vi "Coordinate RND.vi"(8 "error in (no error)":errorcluster, 11 "TSP Class in":refnum<class "TSP Class.lvclass">) -> (0 "error out":errorcluster, 3 "TSP Class out":refnum<class "TSP Class.lvclass">)   [LabVIEW 2015, in "TSP Library.lvlib" / "TSP Class.lvclass"]
uses:
  TSP Class.lvclass
  TSP Class.lvclass/TSP Class.ctl
  TSP Library.lvlib
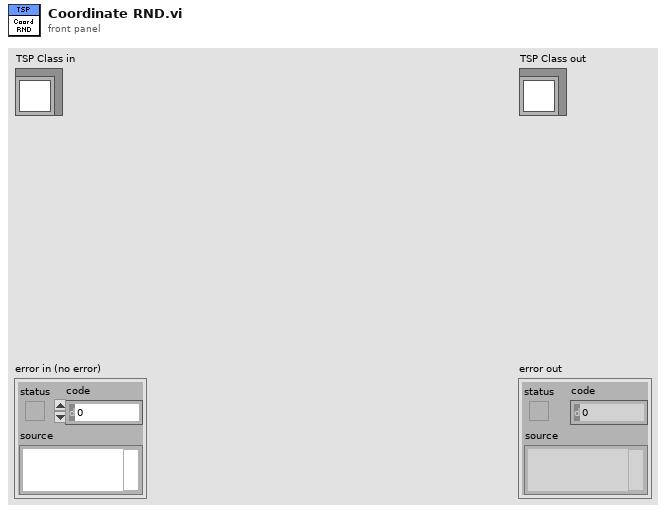
[diagram p1: front panel]
types:
  T1 = typedef "TSP Library.lvlib/Coordinate.ctl" = cluster{"x":dbl, "y":dbl}
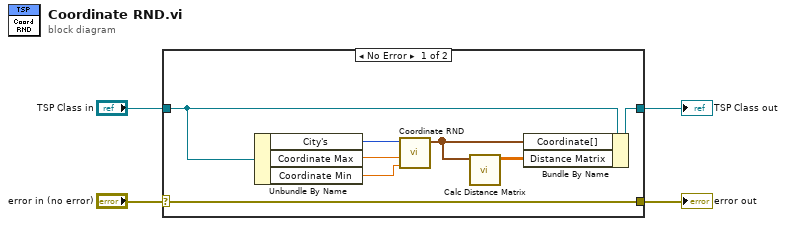
[diagram p0: block diagram]
diagram:
  n1 = case shown="No Error" "error in (no error)" {
    selector: "error in (no error)" -> [w12 w14]
    tunnel: [w12 w14] -> w3
    tunnel: [w11 w13] -> w1
    tunnel: "TSP Class in" -> [w10 w13]
    frame No Error {
      n2 = Unbundle By Name(w10) -> ("City's"=w9:u16, "Coordinate Max"=w7:dbl, "Coordinate Min"=w8:dbl)
      n3 = call "Coordinate RND.vi"("Coordinate Min"=w8, "Coordinate Max"=w7, "City's"=w9) -> ("Coordinate[]"=w5:T1[])  [unwired: 7 in, 1 out]
      n4 = call "Calc Distance Matrix.vi"("Coordinate[] In"=w5) -> ("Distance Matrix"=w6:dbl[][])  [unwired: 10 in]
      n5 = Bundle By Name(cluster=w10, "Coordinate[]"=w5, "Distance Matrix"=w6) -> (w11:refnum<class "TSP Class.lvclass">)
    }
    frame Error {
    }
  }
  "error out" <- w3
  "TSP Class out" <- w1
